vi "noerror.vi"(11 "error in":errorcluster) -> (3 "error out":errorcluster)   [LabVIEW 2015]
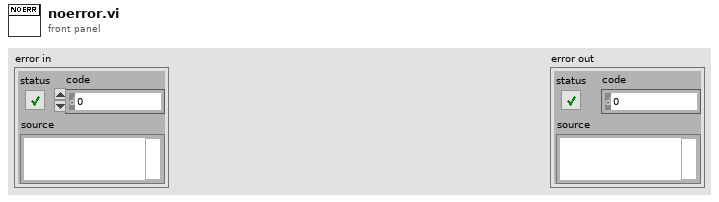
[diagram p1: front panel]
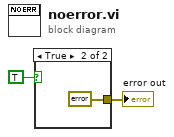
[diagram p0: block diagram]
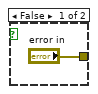
[diagram p2: hidden frame]
diagram:
  n1 = case shown="True" TRUE {
    tunnel: ["error in" errorcluster {"status"=FALSE, "code"=0, "source"=""} ("error out")] -> w1
    frame False {
    }
    frame True {
    }
  }
  "error out" <- w1
